vi "Sensor Data Compiled.vi"() -> ()   [LabVIEW 2019]
panel:
  in  "stop":bool
  out "Table":string[][](table)
  out "Values (STR)":string[](array[string])
  out "Labels":string[](array[string])
  out "data cut":string
  out "error out":errorcluster
  in  "error in":errorcluster
  in  "URL":string="http://www.craigslist.com/sss/"
  out "data":string
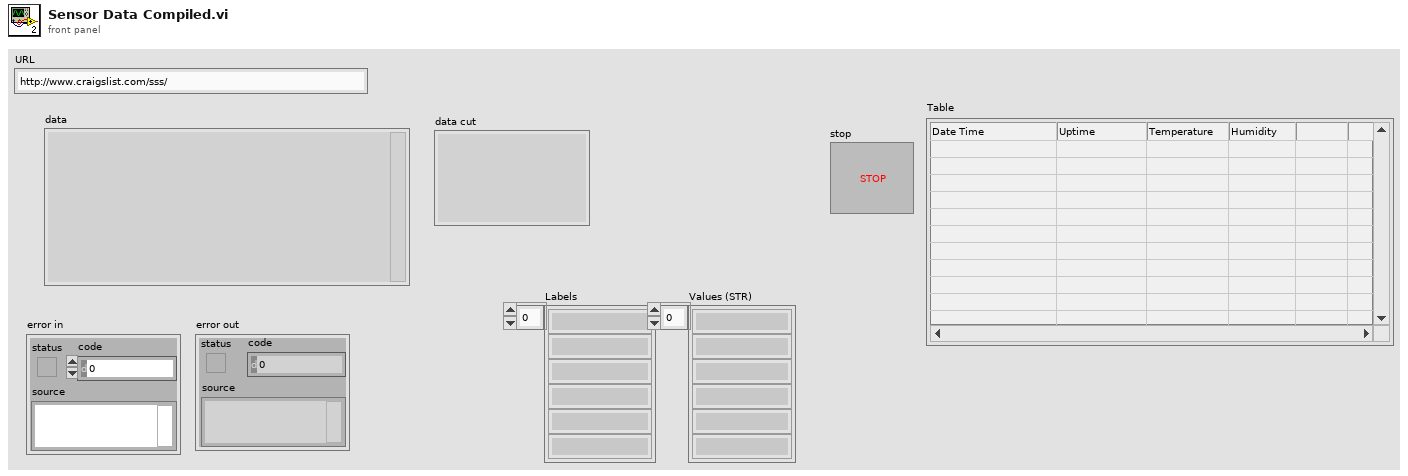
[diagram p1: front panel]
types:
  T1 = enum16{"Read", "Write", "ReadWrite", "BufferedRead", "BufferedReadWrite"}
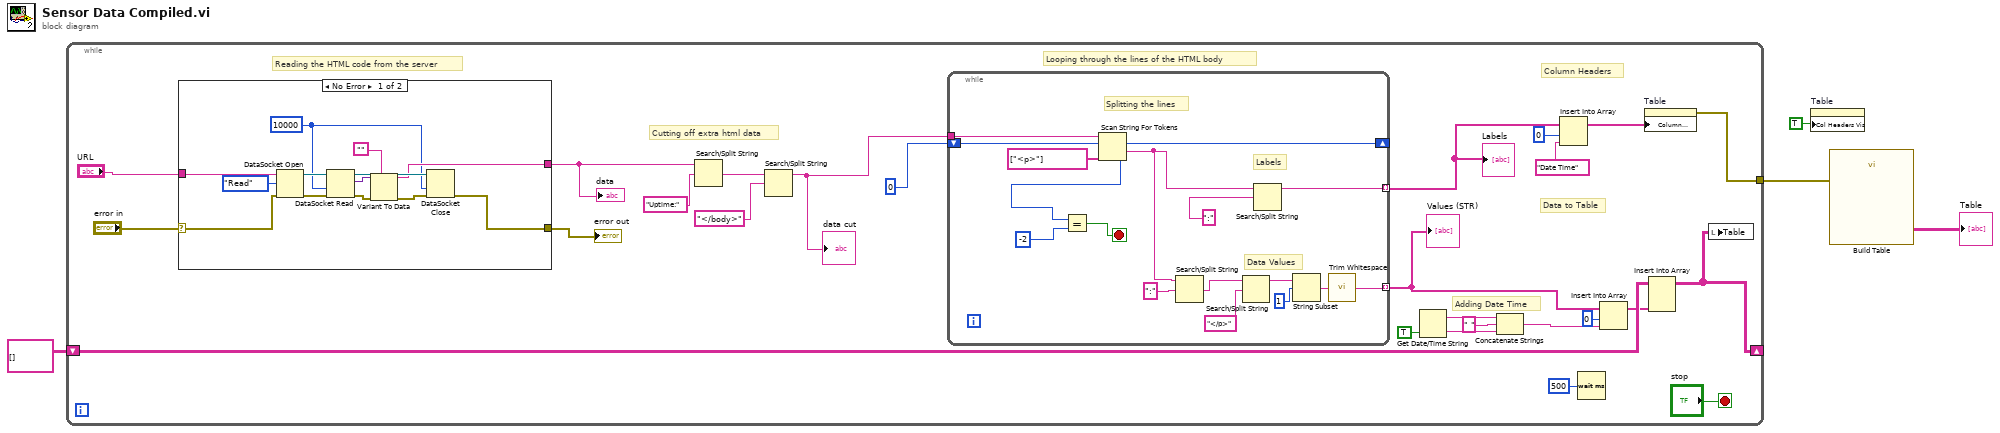
[diagram p0: block diagram]
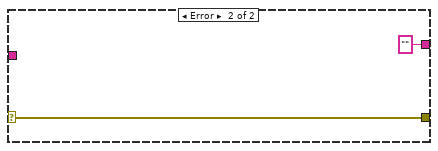
[diagram p2: hidden frame]
diagram:
  n1 = while {
    tunnel: [w21] -> w4
    shift-right: [w14] -> _
    shift-left: string[][] [] -> [w15]
    stop <- "stop" stop-if-true
    # "Adding Date Time"
    # "Data to Table"
    # "Column Headers"
    # "Looping through the lines of the HTML body"
    # "Cutting off extra html data"
    # "Reading the HTML code from the server"
    n2 = case shown="No Error" "error in" {
      selector: "error in" -> [w49 w62]
      tunnel: "URL" -> [w53 _]
      tunnel: [w51 ""] -> w27
      tunnel: [w48 w62] -> w29
      frame No Error {
        w50 = 10000 ("ms timeout (10000)")
        n3 = DataSocket Open(8:w49, 10:T1."Read" ("mode"), 11:w53) -> (0:w57:errorcluster, 3:w60:refnum<k13>)  [unwired: 1 out]
        n4 = DataSocket Read(8:w57, 9:w50, 11:w60) -> (0:w58:errorcluster, 2:w55:variant, 3:w59:refnum<k13>)  [unwired: 2 in, 4 out]
        n5 = Variant To Data(error in=w58, type="", Variant=w55) -> (data=w51:string, error out=w56:errorcluster)
        n6 = DataSocket Close(8:w56, 9:w50, 11:w59) -> (0:w48:errorcluster)  [unwired: 1 out]
      }
      frame Error {
      }
    }
    "data" <- w27
    "error out" <- w29
    n7 = Search/Split String(string=w27, search string/char (-)="Uptime:") -> (match + rest of string=w25:string)  [unwired: 1 in, 2 out]
    n8 = Search/Split String(string=w25, search string/char (-)="</body>") -> (substring before match=w22:string)  [unwired: 1 in, 2 out]
    "data cut" <- w22
    n9 = while {
      shift-right: [w45] -> _
      shift-left: 0 -> [w46]
      tunnel: w22 -> [w47]
      tunnel: [w39] -> w20 mode=indexing
      tunnel: [w34] -> w11 mode=indexing
      stop <- w42 stop-if-true
      # "Data Values"
      # "Labels"
      # "Splitting the lines"
      n10 = Scan String For Tokens(6:string[] ["<p>"] ("delimiters (\\s,\\t,\\r,\\n)"), 8:w46, 9:w47) -> (0:w43:i32, 1:w37:string, 2:w45:i32)  [unwired: 3 in, 1 out]
      n11 = Equal?(x=w43, y=-2) -> (x = y?=w42:bool)
      n12 = Search/Split String(string=w37, search string/char (-)=":") -> (match + rest of string=w35:string)  [unwired: 1 in, 2 out]
      n13 = Search/Split String(string=w35, search string/char (-)="</p>") -> (substring before match=w32:string)  [unwired: 1 in, 2 out]
      n14 = Search/Split String(string=w37, search string/char (-)=":") -> (substring before match=w39:string)  [unwired: 1 in, 2 out]
      n15 = String Subset(string=w32, offset (0)=1) -> (substring=w33:string)  [unwired: 1 in]
      n16 = call <vilib>:"Trim Whitespace.vi"("string"=w33) -> ("trimmed string"=w34:string)  [unwired: 1 in]
    }
    "Labels" <- w20
    "Values (STR)" <- w11
    n17 = Get Date/Time String(want seconds? (F)=TRUE) -> (date string=w6:string, time string=w9:string)  [unwired: 2 in]
    n18 = Concatenate Strings(w6, " " ("string"), w9) -> (w7:string)
    n19 = Insert Into Array(array=w20, index=0, new element="Date Time" ("new element/subarray")) -> (w17:string[])
    n20 = Wait (ms)(milliseconds to wait=u32 500) -> ()  [unwired: 1 out]
    n21 = Insert Into Array(array=w11, index=0, new element=w7) -> (w10:string[])
    n22 = property on="Table" class="Tbl (strict)"("Column Headers[]"=w17) -> (error out=w21:errorcluster)  [unwired: 2 in, 1 out]
    n23 = Insert Into Array(array=w15, new element=w10) -> (w14:string[][])  [unwired: 2 in]
    n24 = local write "Table"(w14) -> ()
  }
  n25 = property on="Table" class="Tbl (strict)"("Col Headers Vis"=TRUE ("Visible Items:Column Headers Visible")) -> ()  [unwired: 2 in, 2 out]
  n26 = call "Build Table"("error in (no error)"=w4) -> ("Table"=→"Table":string[][])  [unwired: 4 in, 6 out]
